vi "FlipFlopTest.vi"() -> ()   [LabVIEW 2012]
uses:
  <vilib>/Waveform/DTblOps.llb/DTbl Boolean Array to Digital.vi
panel:
  out "Digital Waveform Graph 2":digitaldata(graph)
  out "Digital Waveform Graph":digitaldata(graph)
  out "/Q\\":bool
  out "Q":bool
  out "CT":bool
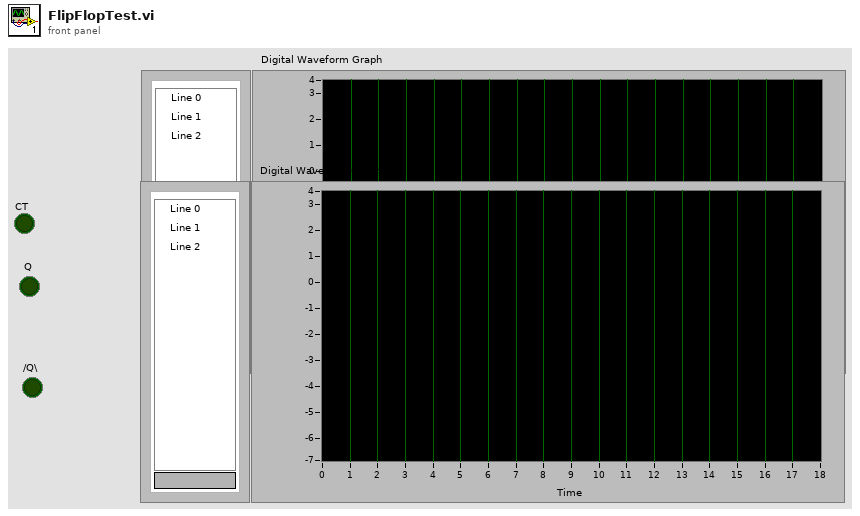
[diagram p1: front panel]
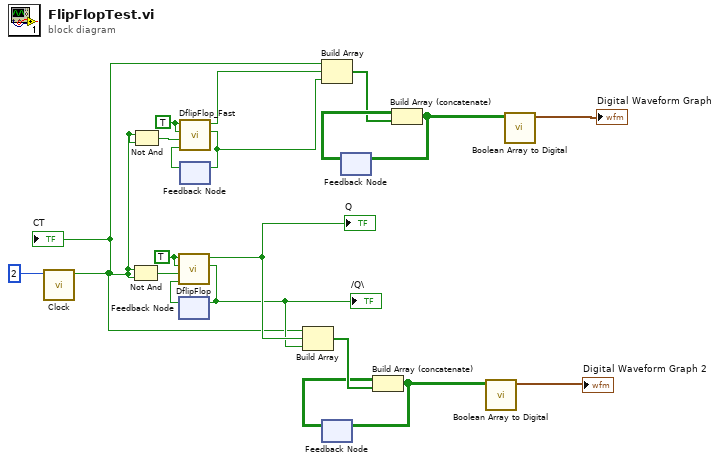
[diagram p0: block diagram]
diagram:
  w9 = TRUE ("Set")
  w19 = TRUE ("Set")
  n1 = call "Clock.vi"("Slices"=u32 2) -> ("Clk"=w3:bool)  [unwired: 10 in]
  "CT" <- w3
  n2 = Not And(1:w3, 2:w3) -> (0:w20:bool)
  n3 = Not And(1:w3, 2:w3) -> (0:w8:bool)
  n4 = feedback #1() -> (w18:bool)  [unwired: 1 in]
  n5 = call "DflipFlop.vi"("D"=w18, "Clock"=w20, "Reset"=w19, "Set"=w19) -> ("/Q\\"=w15:bool, "Q"=w16:bool)  [unwired: 6 in]
  "Q" <- w16
  "/Q\\" <- w15
  n6 = feedback-in #1(w15) -> ()
  n7 = feedback #2() -> (w10:bool)  [unwired: 1 in]
  n8 = call "DflipFlop_Fast.vi"("D"=w10, "Clock"=w8, "Reset"=w9, "Set"=w9) -> ("/Q\\"=w1:bool, "Q"=w2:bool)  [unwired: 6 in]
  n9 = feedback-in #2(w1) -> ()
  n10 = Build Array(w3, w16, w15) -> (w14:bool[])
  n11 = Build Array(w3, w2, w1) -> (w5:bool[])
  n12 = feedback #3() -> (w13:bool[][])  [unwired: 1 in]
  n13 = feedback #4() -> (w6:bool[][])  [unwired: 1 in]
  n14 = Build Array (concatenate)(w13, w14) -> (w12:bool[][])
  n15 = feedback-in #3(w12) -> ()
  n16 = Build Array (concatenate)(w6, w5) -> (w7:bool[][])
  n17 = feedback-in #4(w7) -> ()
  n18 = call-poly <vilib>:"Boolean Array to Digital.vi"("boolean array"=w12) -> ("digital data"=→"Digital Waveform Graph 2":digitaldata)  [unwired: 9 in, 1 out]
  n19 = call-poly <vilib>:"Boolean Array to Digital.vi"("boolean array"=w7) -> ("digital data"=→"Digital Waveform Graph":digitaldata)  [unwired: 9 in, 1 out]
